vi "AssembleBLMultiplotScript-UandTI.vi"(0 "name or relative path":string, 1 "Final Title":string, 2 "Spectra?":bool, 3 "NormaliseHeight?":bool, 4 "Zref":dbl, 5 "Fit Zmax":dbl, 6 "Fit Zmin":dbl, 7 "HeightJitter%":dbl, 8 "Scale":dbl, 9 "BL Targets":T2[](array[typedef]) {"n" min=0.02 max=0.5 step=0.01 format="%.2f"}, 10 "U,L(U)":refnum<vi>, 11 "UtargetsInfo":T1(array[cluster]), 12 "TI,Sigma":refnum<vi>, 13 "TItargetsInfo":T1(array[cluster]), 15 "No d0":cluster{"n":dbl, "d0":dbl, "d0 2":dbl}, 17 "with d0":cluster{"n":dbl, "d0":dbl, "d0 2":dbl}) -> (20 "gnuplotOut":string)   [LabVIEW 2021]
uses:
  BLTarget.ctl
  at.ctl
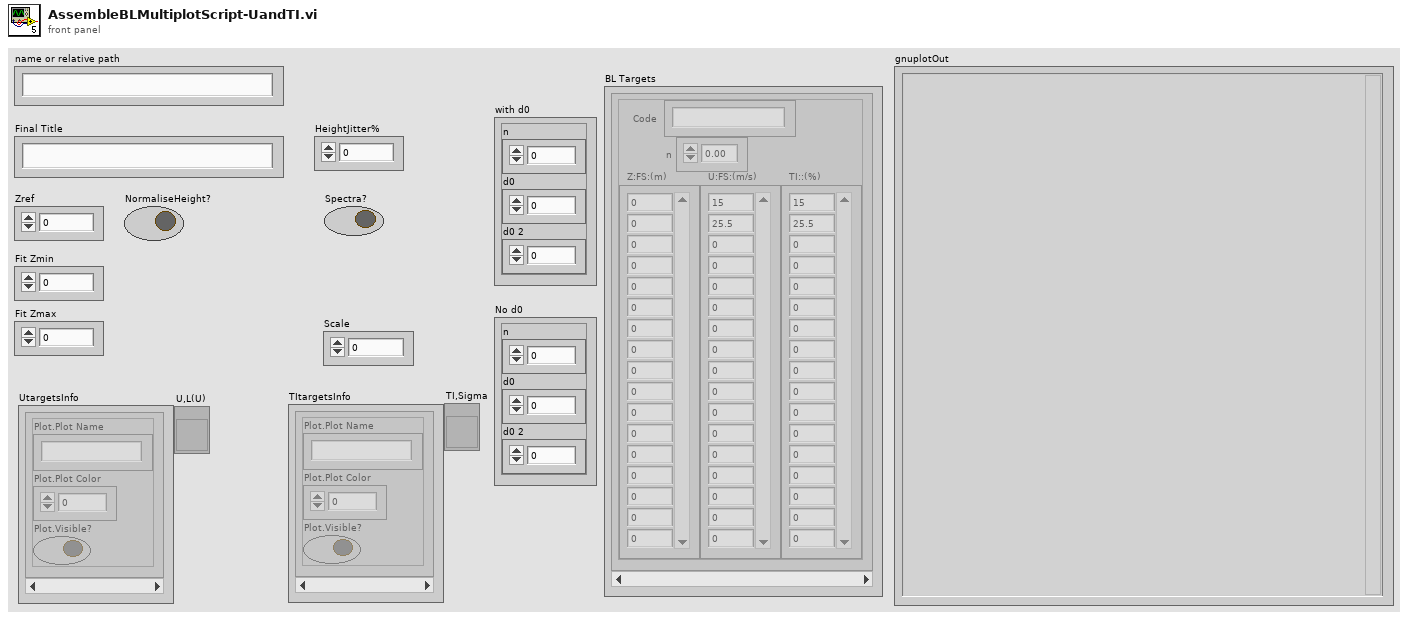
[diagram p1: front panel]
types:
  T1 = cluster{"Plot.Plot Name":string, "Plot.Plot Color":u32, "Plot.Visible?":bool}[]
  T2 = typedef "BLTarget.ctl" = cluster{"Code":string, "n":dbl, "Z:FS:(m)":dbl[], "U:FS:(m/s)":dbl[], "TI::(%)":dbl[]}
  T3 = typedef "at.ctl" = cluster{"XcoordSys":string, "YcoordSys":string, "Xvalue":dbl, "Yvalue":dbl}
  T4 = typedef "minAndMax.ctl" = cluster{"Min":T5, "Max":T5}
  T5 = typedef "AutoManualNumber.ctl" = cluster{"Auto":bool, "Value":dbl}
  T6 = cluster{"No d0":cluster{"n":dbl, "d0":dbl, "d0 2":dbl}, "with d0":cluster{"n":dbl, "d0":dbl, "d0 2":dbl}}
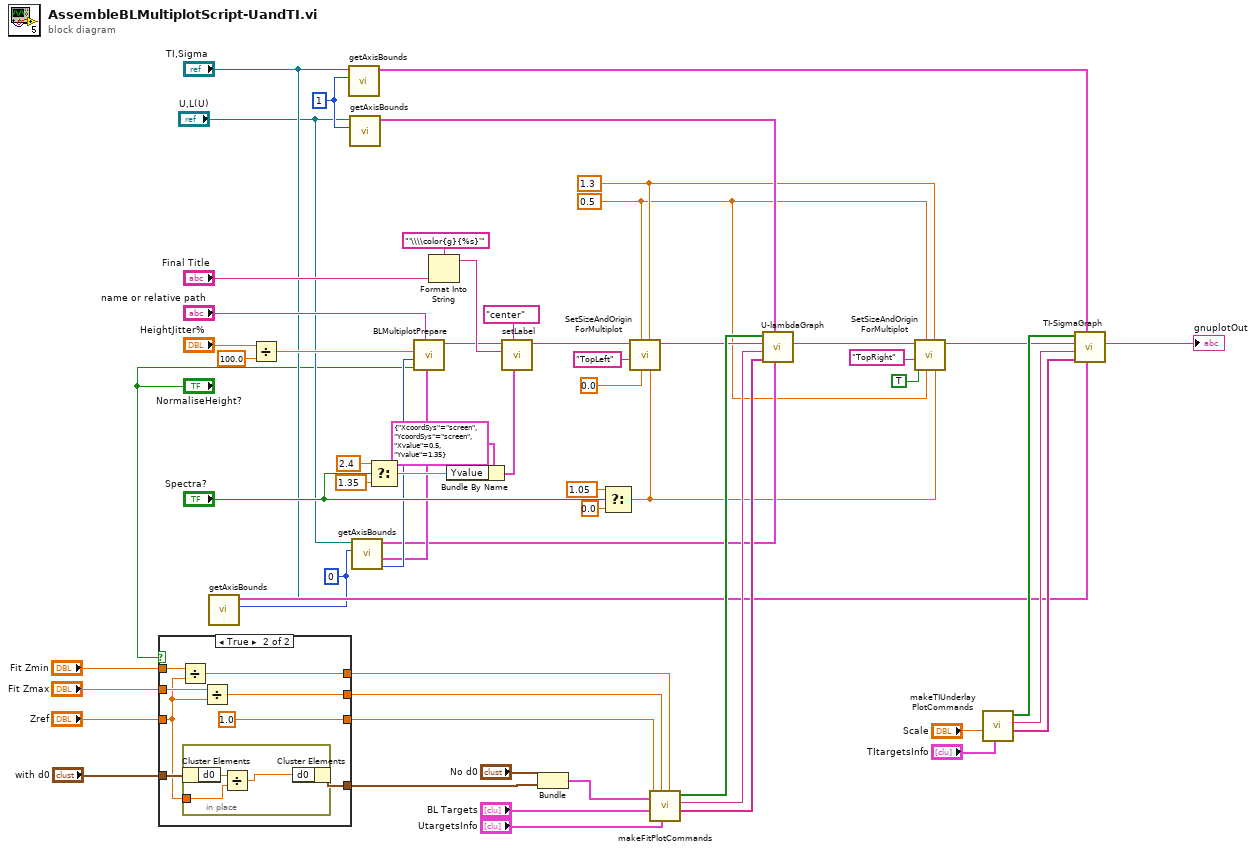
[diagram p0: block diagram]
diagram:
  w18 = 0.5 ("IndividualWidth")
  w19 = 1.3 ("IndividualHeight")
  w13 = 1 ("Active X Scale")
  w12 = 0 ("Active X Scale")
  n1 = case shown="True" "NormaliseHeight?" {
    tunnel: "Fit Zmin" -> [w64 w72]
    tunnel: "Zref" -> [w62 w67]
    tunnel: "Fit Zmax" -> [w63 w71]
    tunnel: [w64 w70] -> w5
    tunnel: [w63 w69] -> w4
    tunnel: [w62 1.0 ("Zref")] -> w3
    tunnel: "with d0" -> [w61 w68]
    tunnel: [w61 w66] -> w1
    frame False {
    }
    frame True {
      n2 = Divide(x=w72, y=w67) -> (x/y=w70:dbl)
      n3 = in-place {
        in-place-border: w67 -> [w74]
        n4 = in-place-cluster #1(w68) -> ("d0"=w75:dbl)
        n5 = Divide(x=w75, y=w74) -> (x/y=w73:dbl)
        n6 = in-place-cluster #1("d0"=w73) -> (w66:cluster{"n":dbl, "d0":dbl, "d0 2":dbl})
      }
      n7 = Divide(x=w71, y=w67) -> (x/y=w69:dbl)
    }
  }
  n8 = call "getAxisBounds.vi"("Active X Scale"=w12, "XYGraph in"="TI,Sigma") -> ("Xbounds"=w29:T4)  [unwired: 6 in, 3 out]
  n9 = Divide(x="HeightJitter%", y=100.0) -> (x/y=w30:dbl)
  n10 = call "getAxisBounds.vi"("Active X Scale"=w13, "XYGraph in"="TI,Sigma") -> ("Xbounds"=w25:T4)  [unwired: 6 in, 3 out]
  n11 = call "getAxisBounds.vi"("Active X Scale"=w13, "XYGraph in"="U,L(U)") -> ("Xbounds"=w27:T4)  [unwired: 6 in, 3 out]
  n12 = call "getAxisBounds.vi"("Active X Scale"=w12, "XYGraph in"="U,L(U)") -> ("YMapping"=w33:enum8{"Lin", "Log"}, "Ybounds"=w32:T4, "Xbounds"=w28:T4)  [unwired: 6 in, 1 out]
  n13 = Select(t=2.4 ("Yvalue"), s="Spectra?", f=1.35 ("Yvalue")) -> (s? t:f=w57:dbl)
  n14 = call "BLMultiplotPrepare.vi"("HeightAxisBounds"=w32, "ProfileFilename"="name or relative path", "NormaliseHeight?"="NormaliseHeight?", "YaxisMapping"=w33, "jitterFraction"=w30) -> ("gnuplotOut"=w35:string)  [unwired: 6 in]
  n15 = Format Into String(format string="'\\\\color{g}{%s}'" ("string"), "Final Title") -> (resulting string=w40:string)  [unwired: 2 in, 1 out]
  n16 = Bundle By Name(cluster=T3 {"XcoordSys"="screen", "YcoordSys"="screen", "Xvalue"=0.5, "Yvalue"=1.35} ("\"At\" location"), "Yvalue"=w57) -> (w53:T3)
  n17 = call "setLabel.vi"("\"At\" location"=w53, "Justify"="center" ("Horizontal"), "singleLabel"=w40, "String in"=w35) -> ("String out"=w36:string)  [unwired: 6 in, 1 out]
  n18 = Bundle("No d0"="No d0", "with d0"=w1) -> (w46:T6)  [unwired: 1 in]
  n19 = Select(t=1.05, s="Spectra?", f=0.0) -> (s? t:f=w26:dbl)
  n20 = call "SetSizeAndOriginForMultiplot.vi"("VerticalPosition"=w26, "Height"=w19, "LateralPosition"=0.0, "Width"=w18, "PlotLocationDescription"="TopLeft", "gnuplotIn"=w36) -> ("gnuplotOut"=w24:string)  [unwired: 5 in]
  n21 = call "makeFitPlotCommands.vi"("Fit Zmin"=w5, "plotInfoArray"="UtargetsInfo", "Fit Zmax"=w4, "BL Targets"="BL Targets", "Coefficients"=w46, "Zref"=w3) -> ("UnderlayPlotSeries"=w42:string[], "Pre-plot Injection"=w41:string, "BasicsVisible"=w59:bool[])  [unwired: 3 in]
  n22 = call "U-lambdaGraph.vi"("U/Uref bounds"=w28, "lambda bounds"=w27, "UnderlayPlotSeries"=w42, "Pre-plot Injection"=w41, "gnuplotIn"=w24, "BasicsVisible"=w59) -> ("gnuplotOut"=w43:string)  [unwired: 5 in]
  n23 = call "SetSizeAndOriginForMultiplot.vi"("VerticalPosition"=w26, "Height"=w19, "LateralPosition"=w18, "Width"=w18, "ClearLabels?"=TRUE, "PlotLocationDescription"="TopRight", "gnuplotIn"=w43) -> ("gnuplotOut"=w20:string)  [unwired: 4 in]
  n24 = call "makeTIUnderlayPlotCommands.vi"("plotInfoArray"="TItargetsInfo", "Scale"="Scale") -> ("UnderlayPlotSeries"=w49:string[], "Pre-plot Injection"=w51:string, "Basics Visible"=w60:bool[])  [unwired: 7 in]
  n25 = call "TI-SigmaGraph.vi"("TI bounds"=w29, "sigma/U bounds"=w25, "UnderlayPlotSeries"=w49, "Pre-plot Injection"=w51, "gnuplotIn"=w20, "Basics Visible"=w60) -> ("gnuplotOut"=→"gnuplotOut":string)  [unwired: 5 in]
